vi "NI Camera Loop.vi"(6 "Used functions":bool=TRUE, 8 "error in":errorcluster, 9 "IBM OptoElectroMechanics Configuration":T1={"Parameter Analizer"={"Parameter Analyzer VISA Session"="COM1", "Sweeping Time Parameters"={"Integration Time"=0, "Short Integration Time (s)"=1.0, "Long Integration Time (s)"=0.0, "Wait Time Parameter"=1.0}, "Acquisition Mode"=enum."Sweeping Mode", "Status Polling Time (ms)"=0, "Comment"="Test VI", "SMU 1 - Sweeping"={"Start / Offset"=0.0, "Stop / Ratio"=1.0, "Step \n(linear only)"=0.01, "Compliance"=0.1, "Power \nCompliance"=0.0, "Mode"=0, "Function"=0, "Sweep Mode"=FALSE}, "SMU 2 - Sweeping"={"Start / Offset"=0.0, "Stop / Ratio"=1.0, "Step \n(linear only)"=0.01, "Compliance"=0.1, "Power \nCompliance"=0.0, "Mode"=0, "Function"=0, "Sweep Mode"=FALSE}, "SMU 3 - Sweeping"={"Start / Offset"=0.0, "Stop / Ratio"=1.0, "Step \n(linear only)"=0.01, "Compliance"=0.1, "Power \nCompliance"=0.0, "Mode"=0, "Function"=0, "Sweep Mode"=FALSE}, "SMU 4 - Sweeping"={"Start / Offset"=0.0, "Stop / Ratio"=1.0, "Step \n(linear only)"=0.01, "Compliance"=0.1, "Power \nCompliance"=0.0, "Mode"=0, "Function"=0, "Sweep Mode"=FALSE}, "Sweep Spacing"=0, "Range"=0, "SMU1 - Sampling"={"Source"=10.0, "Compliance"=1e-05, "Mode"=0, "Function"=FALSE}, "SMU2 - Sampling"={"Source"=1.0, "Compliance"=1.0, "Mode"=0, "Function"=FALSE}, "SMU3 - Sampling"={"Source"=10.0, "Compliance"=1e-05, "Mode"=0, "Function"=FALSE}, "SMU4 - Sampling"={"Source"=0.1, "Compliance"=60.0, "Mode"=10, "Function"=FALSE}, "Sampling Time Parameters"={"Initial Interval (s)"=0.1, "Number of Samples"=60, "Total Sampling Time (s)"=10.0, "Hold Time (s)"=0.0, "Sampling Mode"=0, "Sampling Time"=0}, "Stop Condition"={"Enable Delay (s)"=0.0, "Name"="", "Threshold"=0.0, "num. of events"=1, "Event"=0, "Stop Condition Enable"=FALSE}}, "Switching Matrix"={"Switching Matrix VISA Session"="GPIB0::18::INSTR", "Connections"=[{"Connections"=[FALSE, FALSE, FALSE, FALSE, FALSE, FALSE, FALSE, FALSE, FALSE, FALSE, FALSE, FALSE], "Connection Type"=enum."Disconnected"}, {"Connections"=[FALSE, FALSE, FALSE, FALSE, FALSE, FALSE, FALSE, FALSE, FALSE, FALSE, FALSE, FALSE], "Connection Type"=enum."Disconnected"}, {"Connections"=[FALSE, FALSE, FALSE, FALSE, FALSE, FALSE, FALSE, FALSE, FALSE, FALSE, FALSE, FALSE], "Connection Type"=enum."Disconnected"}, {"Connections"=[FALSE, FALSE, FALSE, FALSE, FALSE, FALSE, FALSE, FALSE, FALSE, FALSE, FALSE, FALSE], "Connection Type"=enum."Disconnected"}, {"Connections"=[FALSE, FALSE, FALSE, FALSE, FALSE, FALSE, FALSE, FALSE, FALSE, FALSE, FALSE, FALSE], "Connection Type"=enum."Disconnected"}, {"Connections"=[FALSE, FALSE, FALSE, FALSE, FALSE, FALSE, FALSE, FALSE, FALSE, FALSE, FALSE, FALSE], "Connection Type"=enum."Disconnected"}, {"Connections"=[FALSE, FALSE, FALSE, FALSE, FALSE, FALSE, FALSE, FALSE, FALSE, FALSE, FALSE, FALSE], "Connection Type"=enum."Disconnected"}, {"Connections"=[FALSE, FALSE, FALSE, FALSE, FALSE, FALSE, FALSE, FALSE, FALSE, FALSE, FALSE, FALSE], "Connection Type"=enum."Disconnected"}]}, "Stress Control"={"Stress Control VISA Session"="StrainMotor", "Axis"=0, "Motion"=0, "Destination (°)"=0.0, "Speed (°/s)"=4.0, "Position (°)"=25.0}, "Optical Spectrometer"={"Laser Settings"={"Laser Wavelength"=enum."365 nm", "Neutral Density Filter"=enum."100%"}, "Spectrometer Settings"={"Confocal Hole Size (µm)"=0.0, "Grating"=2, "Detector"=enum."InGaAs Array"}, "Acquisition Settings"={"Acquisition Mode"=enum."Multi-Window", "Spectal Position (nm)"=632.0, "From (nm)"=735.0, "To (nm)"=0.0, "Integration Time (s)"=0.0, "Number of Accumulations"=3, "AutoScanning"=FALSE, "Spike Removal"=FALSE}, "Path"=path "C:/07 - Prizes and Awards/Marie Curie Prize/Reply Editors Final NCOMMS(10).docx"}, "Switches & Mirrors"={"Relay VISA Session"="COM1", "Switches"={"Laser"=FALSE, "Video"=FALSE}, "Delays (ms)"={"Laser"=500, "Video"=1500}}, "Camera"={"Settings"={"Pixel clock"=20, "Frame rate"=30.0, "Exposure time"=33.21525, "Master Gain"=0, "Red Gain"=0, "Green Gain"=0, "Blue Gain"=0, "Auto Gain"=FALSE, "White-balance"=FALSE, "Color Correction"=FALSE}}, "XYZ Stage"={"Connection Settings"={"Tango VISA"="", "Baudrate"=57600, "Show Protocol?"=FALSE}, "Manual Control"={"North"=FALSE, "South"=FALSE, "West"=FALSE, "East"=FALSE, "Up"=FALSE, "Down"=FALSE, "Stop"=FALSE, "XY Step"=0.0, "Z step"=0.0}, "Coordinate Control"={"Motion Mode"=enum."Absolute", "Destination [mm]"=[]}}, "AutoFocus"={"Matching Criteria"={"Minimum Score"=700.0, "Color Score Weight"=700.0, "Minimum Contrast"=50, "Match Mode"=0, "Match Feature Mode"=0, "Subpixel Accuracy"=TRUE, "Color Sensitivity"=1, "Search Strategy"=1}, "Z Scan Parameters"={"Z Range"=1380.0, "Resolution"=5000.0, "Initial Direction"=enum."Up", "Focus Threshold"=0.1, "Ascent Constant"=0.1}, "Displacement"=0.0, "Transformation Matrix"=[]}, "Sava Data"={"Workspace Info"={"Device Name"="ProberHead_Tst_C29K3_7(2)", "Device Info"="ProberHead_Tst_C29", "Path"=path "C:/Users/gio/Desktop/ProbeHeadTest"}, "Instrument Configuration"={"Instrument"=enum."Unknown Instrument", "Configuration"="Test Configuration"}, "Stress Motor Position"=0.0, "Electrical Measurement"={"Sequence"=[], "V1"=[], "V2"=[], "V3"=[], "V4"=[], "I1"=[], "I2"=[], "I3"=[], "I4"=[]}, "Optical Spectrum"={"Intensity"=[], "Wavelength"=[], "Energy"=[], "Raman Shift"=[], "Detector Temperature"=0.0}}, "PlotData"={"Sliders"={"Strain Sequence"=0, "Instrument Sequence"=0}, "Measurement"={"Which Instrument?"=enum."No Plot", "Electrical Measurement"={"Sequence"=[], "V1"=[], "V2"=[], "V3"=[], "V4"=[], "I1"=[], "I2"=[], "I3"=[], "I4"=[]}, "Measurement Mode"=enum."Sweeping Mode", "Optical Spectrum"={"Intensity"=[], "Wavelength"=[], "Energy"=[], "Raman Shift"=[], "Detector Temperature"=0.0}}, "Instrument Steps"=[], "Strain Points"=[]}, "Instrument Sequence"={"Caller VI"=enum."User"}, "Strain Measurement"={"Stress Sequence "={"Max Motor Position"=1380.0, "# Intermediate Points"=5000, "Initial Direction"=enum."Tension"}, "Track?"=FALSE}} {"AutoFocus"."Displacement" scale=1.0..1000.0; "AutoFocus"."Z Scan Parameters"."Focus Threshold" min=0.0 max=1000.0 step=1.0 format="%#_2f"; "AutoFocus"."Z Scan Parameters"."Ascent Constant" min=0.0 max=1000.0 step=1.0 format="%#_2f"; "AutoFocus"."Z Scan Parameters"."Resolution" min=0.0 max=1.0 step=0.01 format="%_2g"; "AutoFocus"."Z Scan Parameters"."Z Range" format="%_3g"; "AutoFocus"."Matching Criteria"."Match Mode" items=["Shift Invariant", "Rotation Invariant"]; "AutoFocus"."Matching Criteria"."Match Feature Mode" items=["Color and Shape", "Color", "Shape"]; "AutoFocus"."Matching Criteria"."Color Sensitivity" items=["Low Sensitivity", "Medium Sensitivity", "High Sensitivity"]; "AutoFocus"."Matching Criteria"."Search Strategy" items=["Conservative", "Balance", "Aggressive", "Very Aggressive"]; "XYZ Stage"."Manual Control"."Z step" scale=0.1..10.0; "XYZ Stage"."Manual Control"."XY Step" scale=0.1..1000.0; "Camera"."Settings"."Blue Gain" min=0 max=100 scale=0.0..100.0; "Camera"."Settings"."Green Gain" min=0 max=100 scale=0.0..100.0; "Camera"."Settings"."Red Gain" min=0 max=100 scale=0.0..100.0; "Camera"."Settings"."Master Gain" min=0 max=100 scale=0.0..100.0; "Camera"."Settings"."Exposure time" min=0.101625 max=159.246375 step=0.101625 scale=0.101625..159.246375 scale format="%#.3g"; "Camera"."Settings"."Frame rate" min=2.7455631699174137 max=6.2675785993528725 step=0.000101625 scale=2.7455631699174137..6.2675785993528725 scale format="%^#_3g"; "Camera"."Settings"."Pixel clock" min=5 max=43 scale=5.0..43.0; "PlotData"."Sliders"."Instrument Sequence" scale=0.0..10.0; "PlotData"."Sliders"."Strain Sequence" scale=0.0..10.0; "Strain Measurement"."Stress Sequence"."# Intermediate Points" max=1390; "Parameter Analizer"."Stop Condition"."Event" items=["Value > Threshold", "Value < Threshold", "| Value | > | Threshold |", "| Value | < | Threshold |"]; "Parameter Analizer"."Stop Condition"."Threshold" format="%^.2e"; "Parameter Analizer"."Stop Condition"."Enable Delay (s)" format="%.1f"; "Parameter Analizer"."Sampling Time Parameters"."Sampling Time" items=["Auto (linear only)", "No Limit", "Set Limit"]; "Parameter Analizer"."Sampling Time Parameters"."Sampling Mode" items=["Linear", "Log10", "Log25", "Log50", "Thinned Out"]; "Parameter Analizer"."Sampling Time Parameters"."Hold Time (s)" format="%.4f"; "Parameter Analizer"."Sampling Time Parameters"."Total Sampling Time (s)" format="%.1f"; "Parameter Analizer"."Sampling Time Parameters"."Initial Interval (s)" format="%^.3e"; "Parameter Analizer"."SMU 4 - Sweeping"."Function" items=["Disabled", "Var 1", "Var 2", "Var 1'", "Constant"]; "Parameter Analizer"."SMU 4 - Sweeping"."Mode" items=["V", "I", "V pulse", "I  pulse", "Common"]; "Parameter Analizer"."SMU 4 - Sweeping"."Power \nCompliance" format="%^.2e"; "Parameter Analizer"."SMU 4 - Sweeping"."Compliance" format="%^.2e"; "Parameter Analizer"."SMU 4 - Sweeping"."Step \n(linear only)" format="%^.4e"; "Parameter Analizer"."SMU 4 - Sweeping"."Stop / Ratio" format="%^.4e"; "Parameter Analizer"."SMU 4 - Sweeping"."Start / Offset" format="%^.4e"; "Parameter Analizer"."SMU 3 - Sweeping"."Function" items=["Disabled", "Var 1", "Var 2", "Var 1'", "Constant"]; "Parameter Analizer"."SMU 3 - Sweeping"."Mode" items=["V", "I", "V pulse", "I  pulse", "Common"]; "Parameter Analizer"."SMU 3 - Sweeping"."Power \nCompliance" format="%^.2e"; "Parameter Analizer"."SMU 3 - Sweeping"."Compliance" format="%^.2e"; "Parameter Analizer"."SMU 3 - Sweeping"."Step \n(linear only)" format="%^.4e"; "Parameter Analizer"."SMU 3 - Sweeping"."Stop / Ratio" format="%^.4e"; "Parameter Analizer"."SMU 3 - Sweeping"."Start / Offset" format="%^.4e"; "Parameter Analizer"."SMU 2 - Sweeping"."Function" items=["Disabled", "Var 1", "Var 2", "Var 1'", "Constant"]; "Parameter Analizer"."SMU 2 - Sweeping"."Mode" items=["V", "I", "V pulse", "I  pulse", "Common"]; "Parameter Analizer"."SMU 2 - Sweeping"."Power \nCompliance" format="%^.2e"; "Parameter Analizer"."SMU 2 - Sweeping"."Compliance" format="%^.2e"; "Parameter Analizer"."SMU 2 - Sweeping"."Step \n(linear only)" format="%^.4e"; "Parameter Analizer"."SMU 2 - Sweeping"."Stop / Ratio" format="%^.4e"; "Parameter Analizer"."SMU 2 - Sweeping"."Start / Offset" format="%^.4e"; "Parameter Analizer"."SMU 1 - Sweeping"."Function" items=["Disabled", "Var 1", "Var 2", "Var 1'", "Constant"]; "Parameter Analizer"."SMU 1 - Sweeping"."Mode" items=["V", "I", "V pulse", "I  pulse", "Common"]; "Parameter Analizer"."SMU 1 - Sweeping"."Power \nCompliance" format="%^.2e"; "Parameter Analizer"."SMU 1 - Sweeping"."Compliance" format="%^.2e"; "Parameter Analizer"."SMU 1 - Sweeping"."Step \n(linear only)" format="%^.4e"; "Parameter Analizer"."SMU 1 - Sweeping"."Stop / Ratio" format="%^.4e"; "Parameter Analizer"."SMU 1 - Sweeping"."Start / Offset" format="%^.4e"; "Parameter Analizer"."Sweeping Time Parameters"."Long Integration Time (s)" scale=0.02..2.0; "Parameter Analizer"."Sweeping Time Parameters"."Short Integration Time (s)" scale=8e-05..0.00192; "Parameter Analizer"."Sweeping Time Parameters"."Integration Time" items=["Short", "Long"]; "Parameter Analizer"."Sweeping Time Parameters"."Wait Time Parameter" format="%.1f"; "Parameter Analizer"."SMU4 - Sampling"."Mode" items=["V", "I", "Common"]; "Parameter Analizer"."SMU4 - Sampling"."Compliance" format="%^.2e"; "Parameter Analizer"."SMU4 - Sampling"."Source" format="%^.3e"; "Parameter Analizer"."SMU3 - Sampling"."Mode" items=["V", "I", "Common"]; "Parameter Analizer"."SMU3 - Sampling"."Compliance" format="%^.2e"; "Parameter Analizer"."SMU3 - Sampling"."Source" format="%^.3e"; "Parameter Analizer"."SMU2 - Sampling"."Mode" items=["V", "I", "Common"]; "Parameter Analizer"."SMU2 - Sampling"."Compliance" format="%^.2e"; "Parameter Analizer"."SMU2 - Sampling"."Source" format="%^.3e"; "Parameter Analizer"."SMU1 - Sampling"."Mode" items=["V", "I", "Common"]; "Parameter Analizer"."SMU1 - Sampling"."Compliance" format="%^.2e"; "Parameter Analizer"."SMU1 - Sampling"."Source" format="%^.3e"; "Parameter Analizer"."Range" items=["auto", "fixed", "limited"]; "Parameter Analizer"."Sweep Spacing" items=["linear", "log 10", "log 25", "log 50"]; "Stress Control"."Axis" min=1 max=3; "Stress Control"."Position (°)" format="%.6g"; "Stress Control"."Speed (°/s)" min=0.0 max=4.0 format="%.6f"; "Stress Control"."Destination (°)" min=-2000000000.0 max=2000000000.0 format="%.6f"; "Stress Control"."Motion" items=["Absolute", "Relative"]; "Optical Spectrometer"."Spectrometer Settings"."Grating" items=["1800 l/mm", "150 l/mm"]}, 10 "Message Queues out":T57, 11 "Notifiers":T44) -> (0 "error out":errorcluster)   [LabVIEW 2014]
uses:
  support/Message Queue/All Message Queues.ctl
  support/Message Queue/Message Cluster.ctl
  support/Notifiers/Notifiers.ctl
  support/Message Handler Loop Notifiers.ctl
  Hardware Control/Parameter Analyzer/Parameter Analyzer Notifiers.ctl
  Hardware Control/Switching Matrix/Switching Matrix Notifiers.ctl
  Hardware Control/Stress Control/StressControl Notifiers.ctl
  Hardware Control/Spectrometer/Spectrometer Notifiers.ctl
  Hardware Control/Switches and Mirrors/SwitchesMirrors Notifiers.ctl
  Hardware Control/Camera/Camera Notifiers.ctl
  Hardware Control/XYZ Stage/XYZ Notifications.ctl
  Hardware Control/Autofocus/Autofocus Notifiers.ctl
  Measurements/Optoelectronic Measurement/Optoelectronic Notifiers.ctl
  Measurements/Save Data/SaveData Notifiers.ctl
  Measurements/Instrument Sequence/Instrument Sequence Notifiers.ctl
  support/Configuration/Configuration.ctl
  Hardware Control/Parameter Analyzer/Parameter Analyzer Config.ctl
  Hardware Control/Parameter Analyzer/Parameter Analyzer Integration Parameters.ctl
  Hardware Control/Parameter Analyzer/Parameter Analyzer SMU Sweeping.ctl
  Hardware Control/Parameter Analyzer/Parameter Analyzer Sweep Spacing.ctl
  Hardware Control/Parameter Analyzer/Parameter Analyzer SMU Range.ctl
  Hardware Control/Parameter Analyzer/Parameter Analyzer SMU Sampling.ctl
  Hardware Control/Parameter Analyzer/Parameter Analyzer Sampling Parameters.ctl
  Hardware Control/Parameter Analyzer/Parameter Analyzer Stop Sampling Conditions.ctl
  Hardware Control/Switching Matrix/Switching Matrix Config.ctl
  Hardware Control/Stress Control/StressControl Config.ctl
  Hardware Control/Spectrometer/Spectrometer Config.ctl
  Hardware Control/Spectrometer/Laser Settings.ctl
  Hardware Control/Spectrometer/Laser.ctl
  Hardware Control/Spectrometer/Filter.ctl
  Hardware Control/Spectrometer/Grating Detector Settings.ctl
  Hardware Control/Spectrometer/Grating.ctl
  Hardware Control/Spectrometer/Detector.ctl
  Hardware Control/Spectrometer/Acquisition Settings.ctl
  Hardware Control/Switches and Mirrors/SwitchesMirrors Config.ctl
  Hardware Control/Switches and Mirrors/SwitchesMirrors Status.ctl
  Hardware Control/Camera/Camera Config.ctl
  Hardware Control/Camera/Camera Settings.ctl
  Hardware Control/XYZ Stage/XYZ Config.ctl
  Hardware Control/XYZ Stage/XYZ Connection Settings.ctl
  Hardware Control/XYZ Stage/XYZ Stage Control.ctl
  Hardware Control/XYZ Stage/XYZ Coordinate Control.ctl
  Hardware Control/Autofocus/AutoFocus Config.ctl
  Hardware Control/Autofocus/ZScan.ctl
  <vilib>/Analysis/Matrix/Datatypes/RealMatrix.ctl
  Measurements/Save Data/SaveData Config.ctl
  Measurements/Save Data/SaveData Workspace Info.ctl
  Measurements/Save Data/SaveData Instrument Configuration.ctl
  Measurements/Instrument Sequence/Instrument List.ctl
  Hardware Control/Spectrometer/Spectral Data.ctl
  Measurements/Plot Data/PlotData Config.ctl
  Measurements/Plot Data/Measurement.ctl
  Measurements/Plot Data/WhichInstrument.ctl
  Hardware Control/Parameter Analyzer/Electrical Data.ctl
  Measurements/Instrument Sequence/Instrument Steps.ctl
  Measurements/Instrument Sequence/Action.ctl
  Measurements/Instrument Sequence/Instrument Sequence Config.ctl
  Measurements/Strain Measurement/Strain Measurement Config.ctl
  Hardware Control/Camera/NI Camera Functions.ctl
  support/Message Queue/Message Queue.lvlib
  <vilib>/Analysis/Matrix/NI_Matrix.lvlib
panel:
  # "LICENSED MATERIALS – PROPERTY OF IBM\nCopyright IBM Corp. 2016,\nALL RIGHTS RESERVED"
  # "XY"
  # "Z"
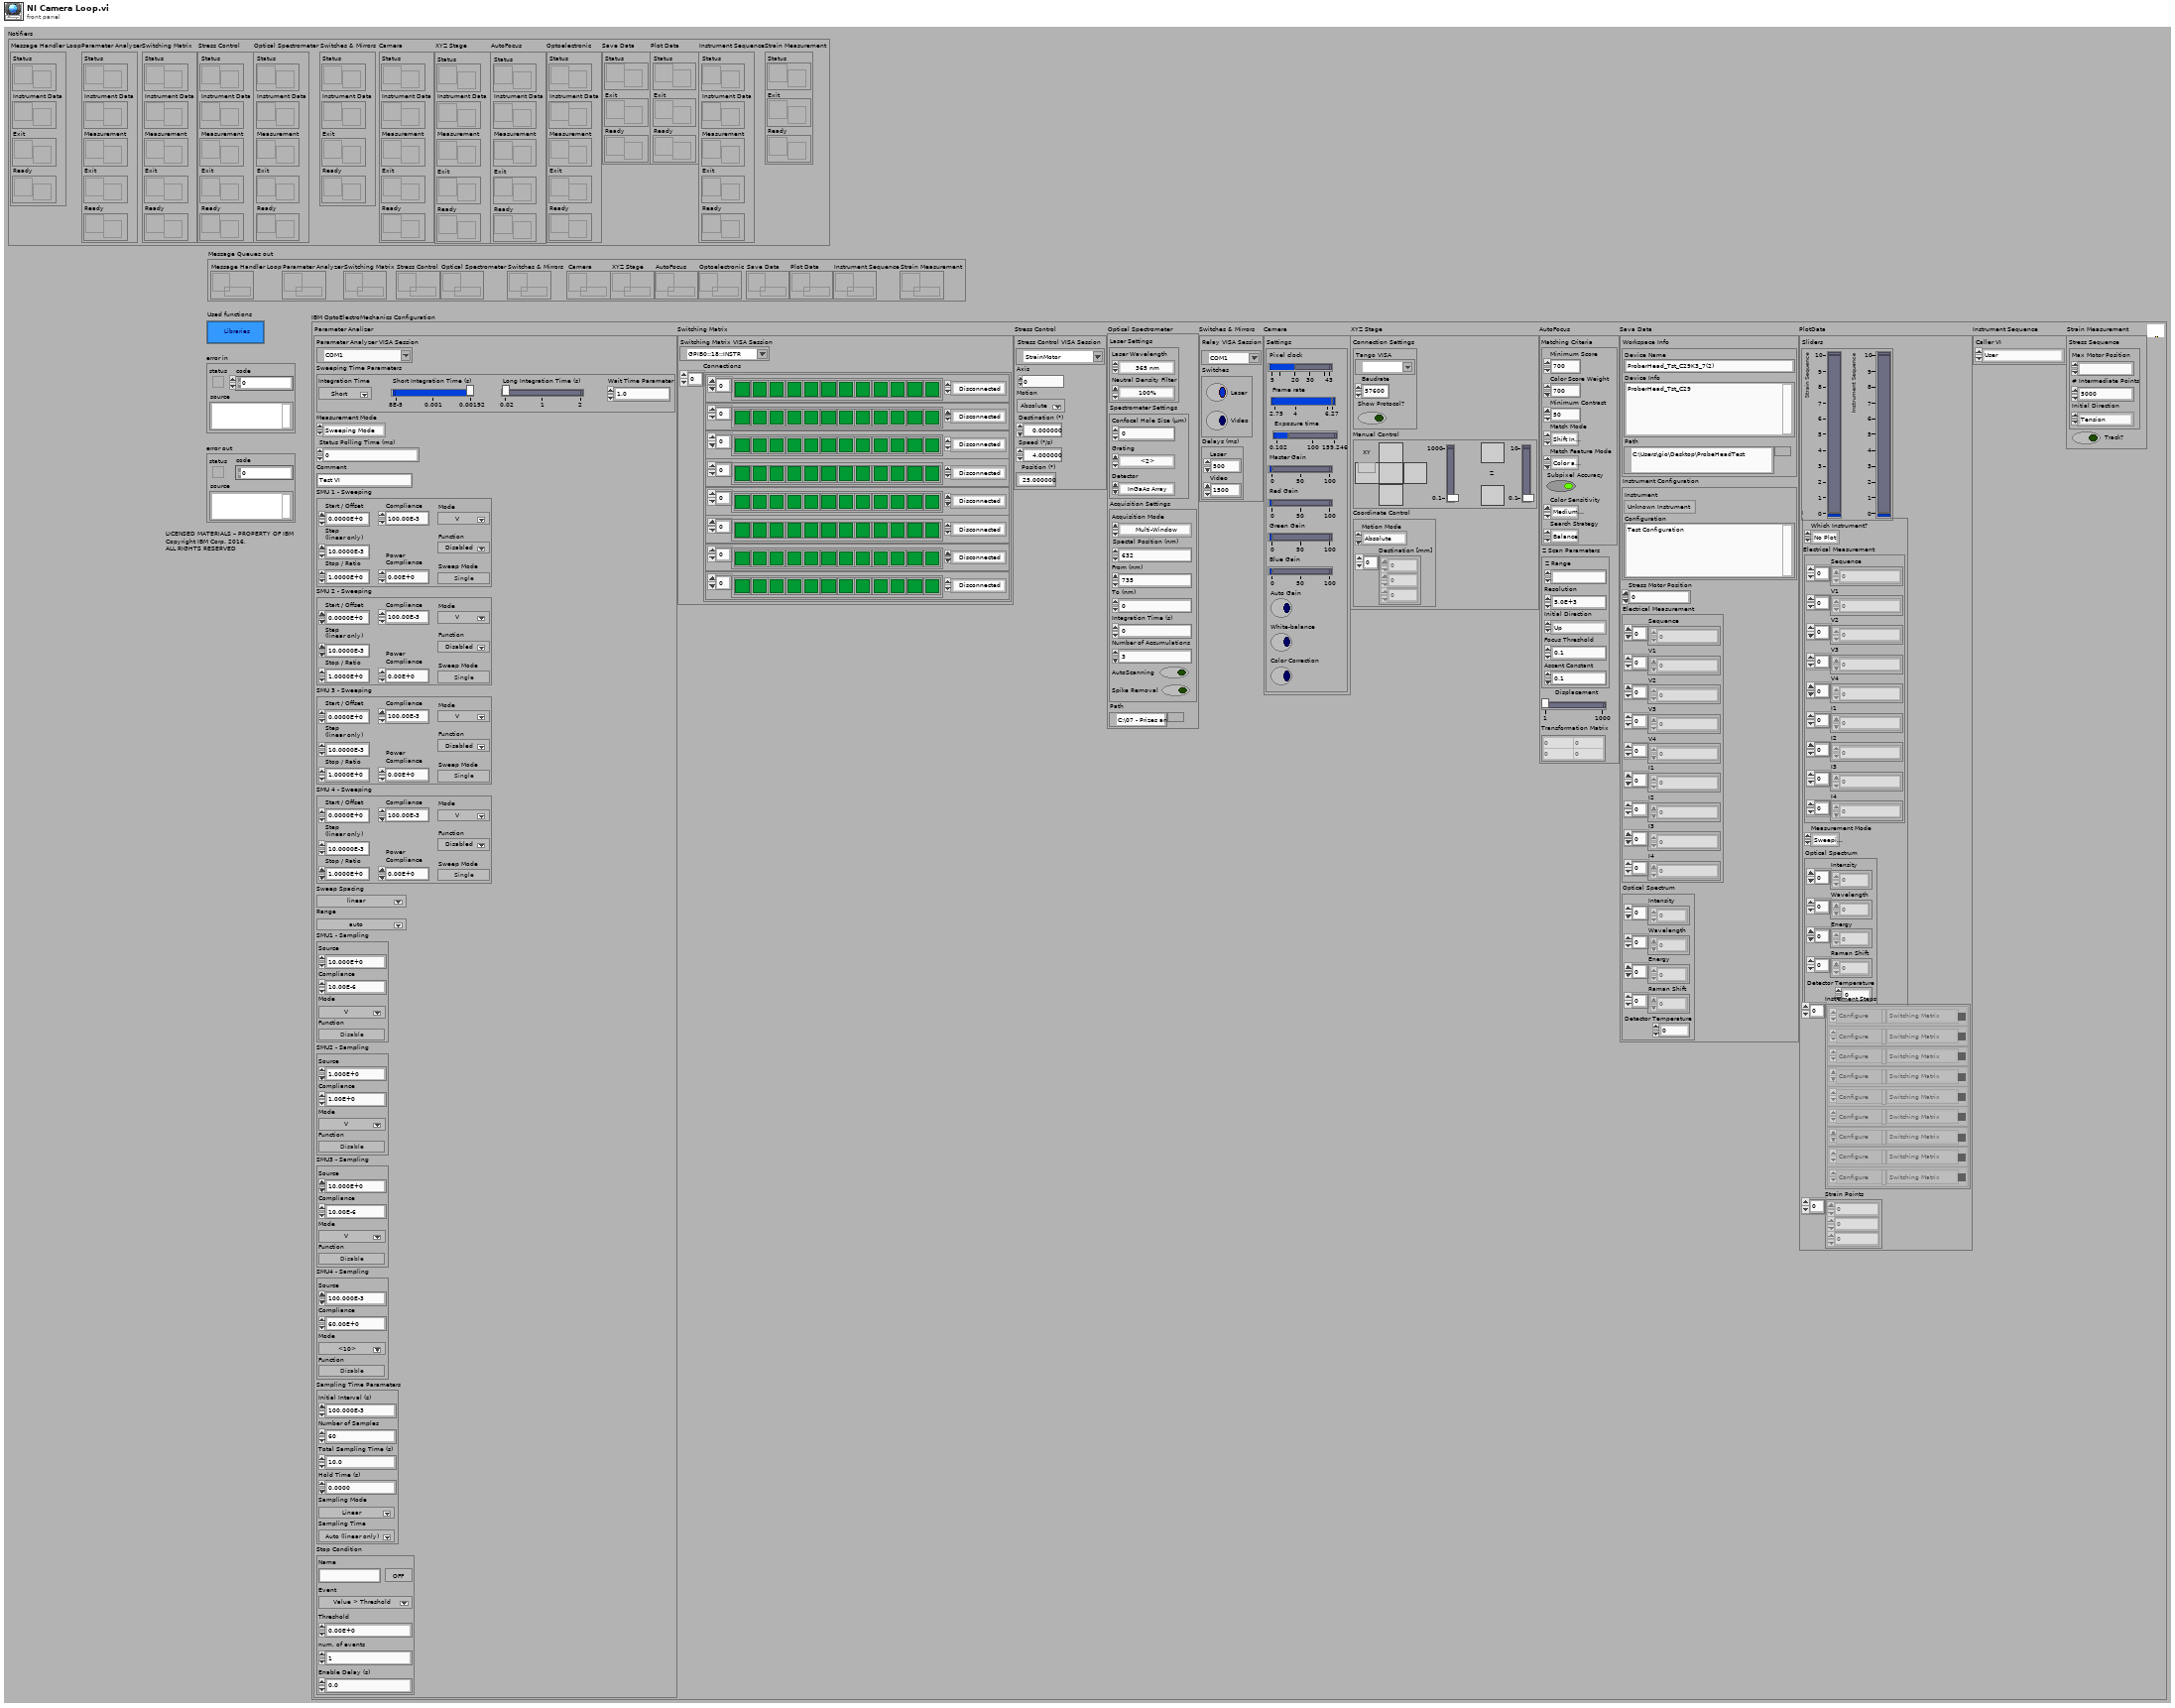
[diagram p1: front panel]
types:
  T1 = typedef "Configuration.ctl" = cluster{"Parameter Analizer":T2, "Switching Matrix":T10, "Stress Control":T11, "Optical Spectrometer":T12, "Switches & Mirrors":T20, "Camera":T22, "XYZ Stage":T24, "AutoFocus":T28, "Sava Data":T31, "PlotData":T36, "Instrument Sequence":T42, "Strain Measurement":T43}
  T2 = typedef "Parameter Analyzer Config.ctl" = cluster{"Parameter Analyzer VISA Session":refnum<visa-resource-name>, "Sweeping Time Parameters":T3, "Acquisition Mode":enum32{"Sweeping Mode", "Sampling Mode"}, "Status Polling Time (ms)":u32, "Comment":string, "SMU 1 - Sweeping":T4, "SMU 2 - Sweeping":T4, "SMU 3 - Sweeping":T4, "SMU 4 - Sweeping":T4, "Sweep Spacing":T5, "Range":T6, "SMU1 - Sampling":T7, "SMU2 - Sampling":T7, "SMU3 - Sampling":T7, "SMU4 - Sampling":T7, "Sampling Time Parameters":T8, "Stop Condition":T9}
  T3 = typedef "Parameter Analyzer Integration Parameters.ctl" = cluster{"Integration Time":u32, "Short Integration Time (s)":dbl, "Long Integration Time (s)":dbl, "Wait Time Parameter":dbl}
  T4 = typedef "Parameter Analyzer SMU Sweeping.ctl" = cluster{"Start / Offset":dbl, "Stop / Ratio":dbl, "Step \n(linear only)":dbl, "Compliance":dbl, "Power \nCompliance":dbl, "Mode":u32, "Function":i32, "Sweep Mode":bool}
  T5 = typedef "Parameter Analyzer Sweep Spacing.ctl" = u16
  T6 = typedef "Parameter Analyzer SMU Range.ctl" = u16
  T7 = typedef "Parameter Analyzer SMU Sampling.ctl" = cluster{"Source":dbl, "Compliance":dbl, "Mode":u32, "Function":bool}
  T8 = typedef "Parameter Analyzer Sampling Parameters.ctl" = cluster{"Initial Interval (s)":dbl, "Number of Samples":i32, "Total Sampling Time (s)":dbl, "Hold Time (s)":dbl, "Sampling Mode":i32, "Sampling Time":i32}
  T9 = typedef "Parameter Analyzer Stop Sampling Conditions.ctl" = cluster{"Enable Delay (s)":dbl, "Name":string, "Threshold":dbl, "num. of events":i32, "Event":i32, "Stop Condition Enable":bool}
  T10 = typedef "Switching Matrix Config.ctl" = cluster{"Switching Matrix VISA Session":refnum<visa-resource-name>, "Connections":cluster{"Connections":bool[], "Connection Type":enum16{"Disconnected", "Make - Break", "Break - Make"}}[]}
  T11 = typedef "StressControl Config.ctl" = cluster{"Stress Control VISA Session":refnum<visa-resource-name>, "Axis":i32, "Motion":u16, "Destination (°)":dbl, "Speed (°/s)":dbl, "Position (°)":dbl}
  T12 = typedef "Spectrometer Config.ctl" = cluster{"Laser Settings":T13, "Spectrometer Settings":T16, "Acquisition Settings":T19, "Path":path}
  T13 = typedef "Laser Settings.ctl" = cluster{"Laser Wavelength":T14, "Neutral Density Filter":T15}
  T14 = typedef "Laser.ctl" = enum16{"633 nm", "784 nm", "532 nm", "365 nm"}
  T15 = typedef "Filter.ctl" = enum16{"100%", "50%", "25%", "10%", "1%", "0.1%", "0.01%"}
  T16 = typedef "Grating Detector Settings.ctl" = cluster{"Confocal Hole Size (µm)":dbl, "Grating":T17, "Detector":T18}
  T17 = typedef "Grating.ctl" = u16
  T18 = typedef "Detector.ctl" = enum16{"InGaAs Array", "Silicon CCD"}
  T19 = typedef "Acquisition Settings.ctl" = cluster{"Acquisition Mode":enum16{"Single Window", "Multi-Window"}, "Spectal Position (nm)":dbl, "From (nm)":dbl, "To (nm)":dbl, "Integration Time (s)":dbl, "Number of Accumulations":i32, "AutoScanning":bool, "Spike Removal":bool}
  T20 = typedef "SwitchesMirrors Config.ctl" = cluster{"Relay VISA Session":refnum<visa-resource-name>, "Switches":T21, "Delays (ms)":cluster{"Laser":u32, "Video":u32}}
  T21 = typedef "SwitchesMirrors Status.ctl" = cluster{"Laser":bool, "Video":bool}
  T22 = typedef "Camera Config.ctl" = cluster{"Settings":T23}
  T23 = typedef "Camera Settings.ctl" = cluster{"Pixel clock":i32, "Frame rate":dbl, "Exposure time":dbl, "Master Gain":i32, "Red Gain":i32, "Green Gain":i32, "Blue Gain":i32, "Auto Gain":bool, "White-balance":bool, "Color Correction":bool}
  T24 = typedef "XYZ Config.ctl" = cluster{"Connection Settings":T25, "Manual Control":T26, "Coordinate Control":T27}
  T25 = typedef "XYZ Connection Settings.ctl" = cluster{"Tango VISA":refnum<visa-resource-name>, "Baudrate":i32, "Show Protocol?":bool}
  T26 = typedef "XYZ Stage Control.ctl" = cluster{"North":bool, "South":bool, "West":bool, "East":bool, "Up":bool, "Down":bool, "Stop":bool, "XY Step":dbl, "Z step":dbl}
  T27 = typedef "XYZ Coordinate Control.ctl" = cluster{"Motion Mode":enum16{"Absolute", "Relative"}, "Destination [mm]":dbl[]}
  T28 = typedef "AutoFocus Config.ctl" = cluster{"Matching Criteria":cluster{"Minimum Score":sgl, "Color Score Weight":sgl, "Minimum Contrast":i32, "Match Mode":u32, "Match Feature Mode":u32, "Subpixel Accuracy":bool, "Color Sensitivity":u32, "Search Strategy":u32}, "Z Scan Parameters":T29, "Displacement":dbl, "Transformation Matrix":T30}
  T29 = typedef "ZScan.ctl" = cluster{"Z Range":ext, "Resolution":dbl, "Initial Direction":enum16{"Up", "Down"}, "Focus Threshold":dbl, "Ascent Constant":dbl}
  T30 = typedef "NI_Matrix.lvlib/RealMatrix.ctl" = dbl[][]
  T31 = typedef "SaveData Config.ctl" = cluster{"Workspace Info":T32, "Instrument Configuration":T33, "Stress Motor Position":dbl, "Electrical Measurement":cluster{"Sequence":dbl[], "V1":dbl[], "V2":dbl[], "V3":dbl[], "V4":dbl[], "I1":dbl[], "I2":dbl[], "I3":dbl[], "I4":dbl[]}, "Optical Spectrum":T35}
  T32 = typedef "SaveData Workspace Info.ctl" = cluster{"Device Name":string, "Device Info":string, "Path":path}
  T33 = typedef "SaveData Instrument Configuration.ctl" = cluster{"Instrument":T34, "Configuration":string}
  T34 = typedef "Instrument List.ctl" = enum32{"Unknown Instrument", "Switching Matrix", "Parameter Analyzer", "Optical Spectrometer", "Optoelectronic", "Autofocus"}
  T35 = typedef "Spectral Data.ctl" = cluster{"Intensity":dbl[], "Wavelength":dbl[], "Energy":dbl[], "Raman Shift":dbl[], "Detector Temperature":dbl}
  T36 = typedef "PlotData Config.ctl" = cluster{"Sliders":cluster{"Strain Sequence":i32, "Instrument Sequence":i32}, "Measurement":T37, "Instrument Steps":T40, "Strain Points":dbl[]}
  T37 = typedef "Measurement.ctl" = cluster{"Which Instrument?":T38, "Electrical Measurement":T39, "Measurement Mode":enum16{"Sweeping Mode", "Sampling Mode"}, "Optical Spectrum":T35}
  T38 = typedef "WhichInstrument.ctl" = enum16{"No Plot", "Spectrometer", "Parameter Analyzer", "Optoelectronic"}
  T39 = typedef "Electrical Data.ctl" = cluster{"Sequence":dbl[], "V1":dbl[], "V2":dbl[], "V3":dbl[], "V4":dbl[], "I1":dbl[], "I2":dbl[], "I3":dbl[], "I4":dbl[]}
  T40 = typedef "Instrument Steps.ctl" = cluster{"Action":T41, "Configuration":variant, "Instrument":T34, "Status":enum8{"False", "True", "Mixed"}}[]
  T41 = typedef "Action.ctl" = enum32{"Configure", "Measure"}
  T42 = typedef "Instrument Sequence Config.ctl" = cluster{"Caller VI":enum16{"User", "Stress Measurement VI"}}
  T43 = typedef "Strain Measurement Config.ctl" = cluster{"Stress Sequence ":cluster{"Max Motor Position":ext, "# Intermediate Points":u32, "Initial Direction":enum16{"Tension", "Compression"}}, "Track?":bool}
  T44 = typedef "Notifiers.ctl" = cluster{"Message Handler Loop":T45, "Parameter Analyzer":T46, "Switching Matrix":T47, "Stress Control":T48, "Optical Spectrometer":T49, "Switches & Mirrors":T50, "Camera":T51, "XYZ Stage":T52, "AutoFocus":T53, "Optoelectronic":T54, "Save Data":T55, "Plot Data":T55, "Instrument Sequence":T56, "Strain Measurement":cluster{"Status":refnum<notifier>, "Exit":refnum<notifier>, "Ready":refnum<notifier>}}
  T45 = typedef "Message Handler Loop Notifiers.ctl" = cluster{"Status":refnum<notifier>, "Instrument Data":refnum<notifier>, "Exit":refnum<notifier>, "Ready":refnum<notifier>}
  T46 = typedef "Parameter Analyzer Notifiers.ctl" = cluster{"Status":refnum<notifier>, "Instrument Data":refnum<notifier>, "Measurement":refnum<notifier>, "Exit":refnum<notifier>, "Ready":refnum<notifier>}
  T47 = typedef "Switching Matrix Notifiers.ctl" = cluster{"Status":refnum<notifier>, "Instrument Data":refnum<notifier>, "Measurement":refnum<notifier>, "Exit":refnum<notifier>, "Ready":refnum<notifier>}
  T48 = typedef "StressControl Notifiers.ctl" = cluster{"Status":refnum<notifier>, "Instrument Data":refnum<notifier>, "Measurement":refnum<notifier>, "Exit":refnum<notifier>, "Ready":refnum<notifier>}
  T49 = typedef "Spectrometer Notifiers.ctl" = cluster{"Status":refnum<notifier>, "Instrument Data":refnum<notifier>, "Measurement":refnum<notifier>, "Exit":refnum<notifier>, "Ready":refnum<notifier>}
  T50 = typedef "SwitchesMirrors Notifiers.ctl" = cluster{"Status":refnum<notifier>, "Instrument Data":refnum<notifier>, "Exit":refnum<notifier>, "Ready":refnum<notifier>}
  T51 = typedef "Camera Notifiers.ctl" = cluster{"Status":refnum<notifier>, "Instrument Data":refnum<notifier>, "Measurement":refnum<notifier>, "Exit":refnum<notifier>, "Ready":refnum<notifier>}
  T52 = typedef "XYZ Notifications.ctl" = cluster{"Status":refnum<notifier>, "Instrument Data":refnum<notifier>, "Measurement":refnum<notifier>, "Exit":refnum<notifier>, "Ready":refnum<notifier>}
  T53 = typedef "Autofocus Notifiers.ctl" = cluster{"Status":refnum<notifier>, "Instrument Data":refnum<notifier>, "Measurement":refnum<notifier>, "Exit":refnum<notifier>, "Ready":refnum<notifier>}
  T54 = typedef "Optoelectronic Notifiers.ctl" = cluster{"Status":refnum<notifier>, "Instrument Data":refnum<notifier>, "Measurement":refnum<notifier>, "Exit":refnum<notifier>, "Ready":refnum<notifier>}
  T55 = typedef "SaveData Notifiers.ctl" = cluster{"Status":refnum<notifier>, "Exit":refnum<notifier>, "Ready":refnum<notifier>}
  T56 = typedef "Instrument Sequence Notifiers.ctl" = cluster{"Status":refnum<notifier>, "Instrument Data":refnum<notifier>, "Measurement":refnum<notifier>, "Exit":refnum<notifier>, "Ready":refnum<notifier>}
  T57 = typedef "Message Queue.lvlib/All Message Queues.ctl" = cluster{"Message Handler Loop":refnum<queue>, "Parameter Analyzer":refnum<queue>, "Switching Matrix":refnum<queue>, "Stress Control":refnum<queue>, "Optical Spectrometer":refnum<queue>, "Switches & Mirrors":refnum<queue>, "Camera":refnum<queue>, "XYZ Stage":refnum<queue>, "AutoFocus":refnum<queue>, "Optoelectronic":refnum<queue>, "Save Data":refnum<queue>, "Plot Data":refnum<queue>, "Instrument Sequence":refnum<queue>, "Strain Measurement":refnum<queue>}
  T58 = typedef "Camera Data.ctl" = cluster{"Configuration":T22, "Refnums":T59, "Initialization":T60}
  T59 = typedef "Camera Refnums.ctl" = cluster{"Pixel Clock":refnum<vi>, "Frame Rate":refnum<vi>, "Exposure Time":refnum<vi>, "Master Gain":refnum<vi>, "Red Gain":refnum<vi>, "Green Gain":refnum<vi>, "Blue Gain":refnum<vi>, "Auto Gain":refnum<vi>, "Auto White-balance":refnum<vi>, "Color Correction":refnum<vi>, "Image":refnum<vi>, "Video Button":refnum<vi>, "Instrument Status":refnum<vi>}
  T60 = typedef "Camera Initialization.ctl" = cluster{"Connect":bool, "Update Refnums":bool, "Acquiring?":bool}
  T61 = typedef "NI Camera Functions.ctl" = enum16{"Connect", "Disconnect", "Start Live", "Stop Live", "Acquire", "Update Refnums"}
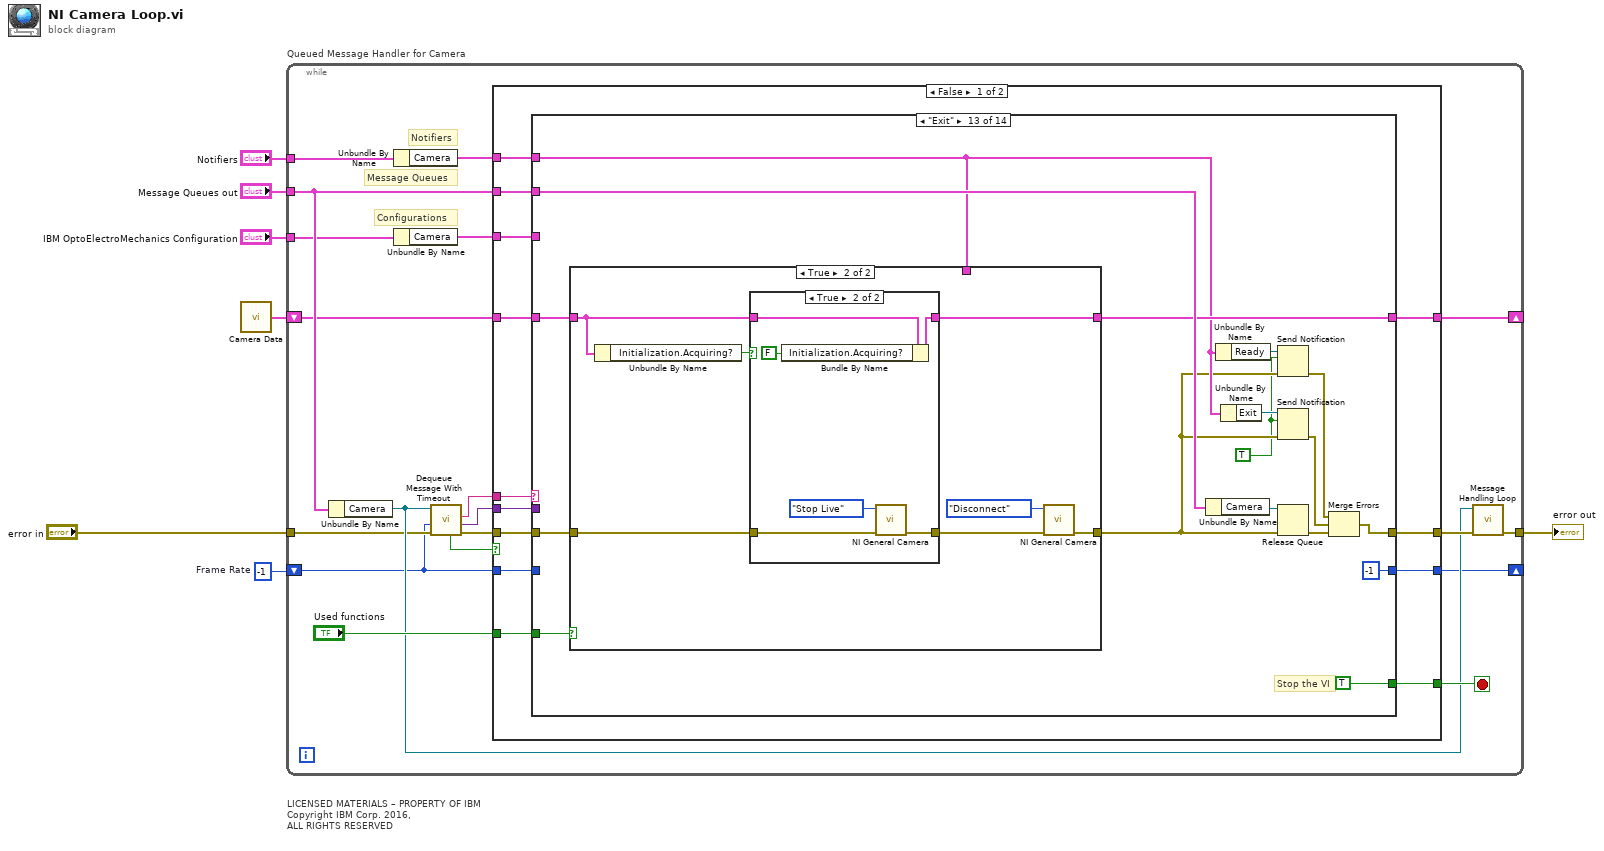
[diagram p0: block diagram]
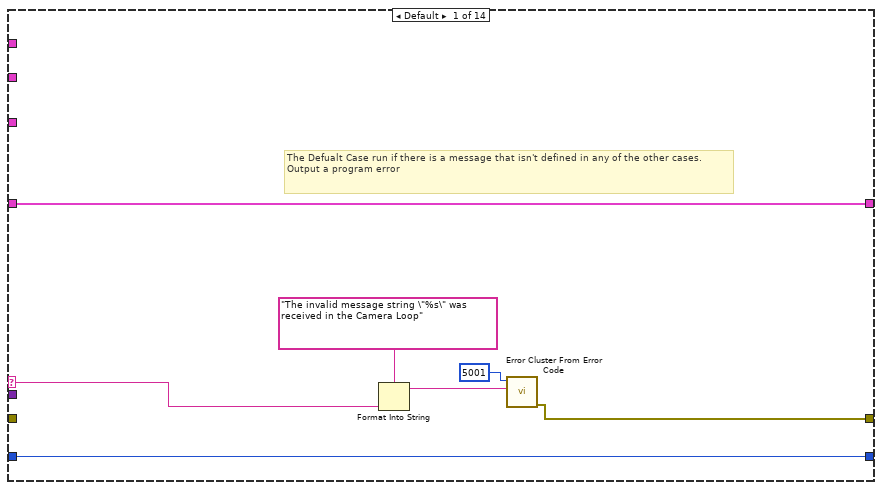
[diagram p2: hidden frame]
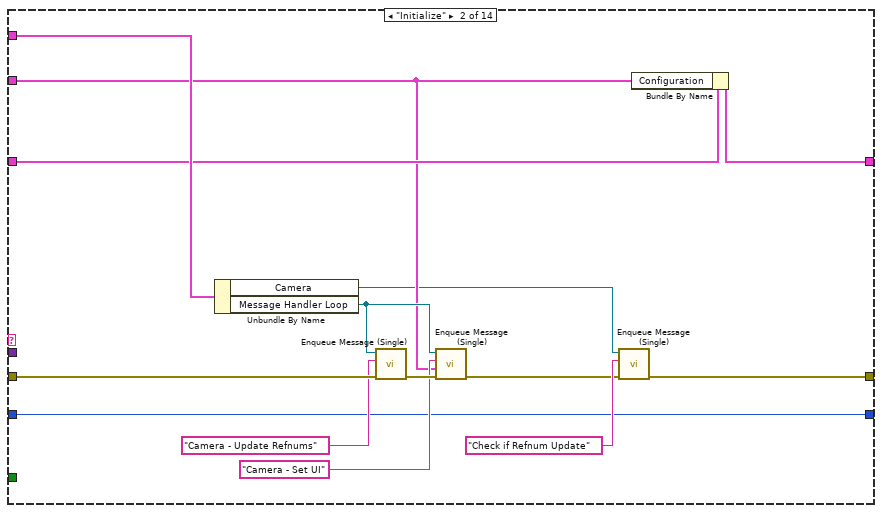
[diagram p3: hidden frame]
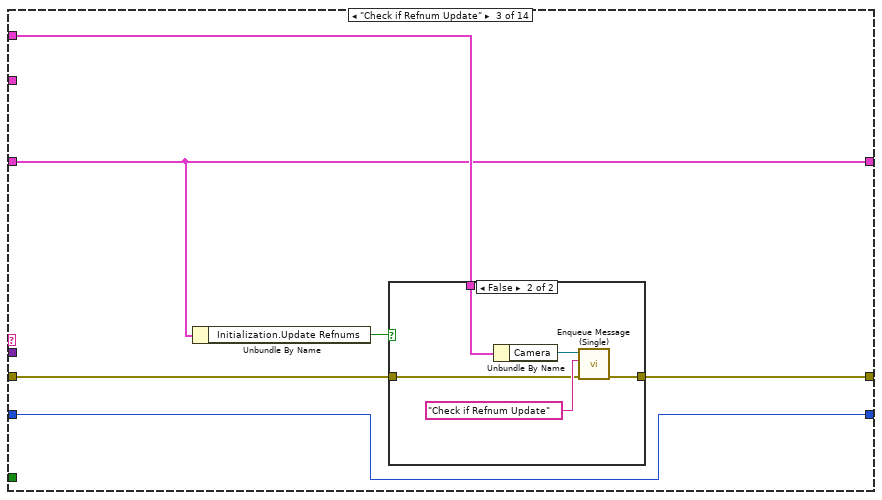
[diagram p4: hidden frame]
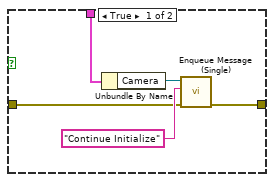
[diagram p5: hidden frame]
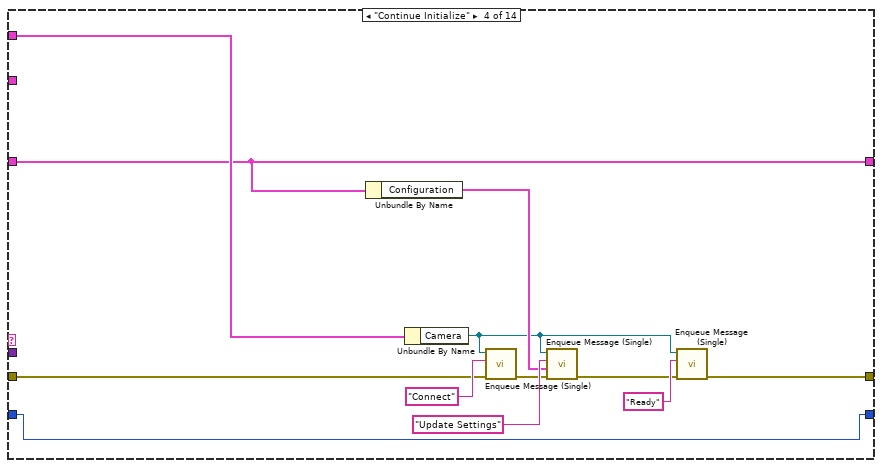
[diagram p6: hidden frame]
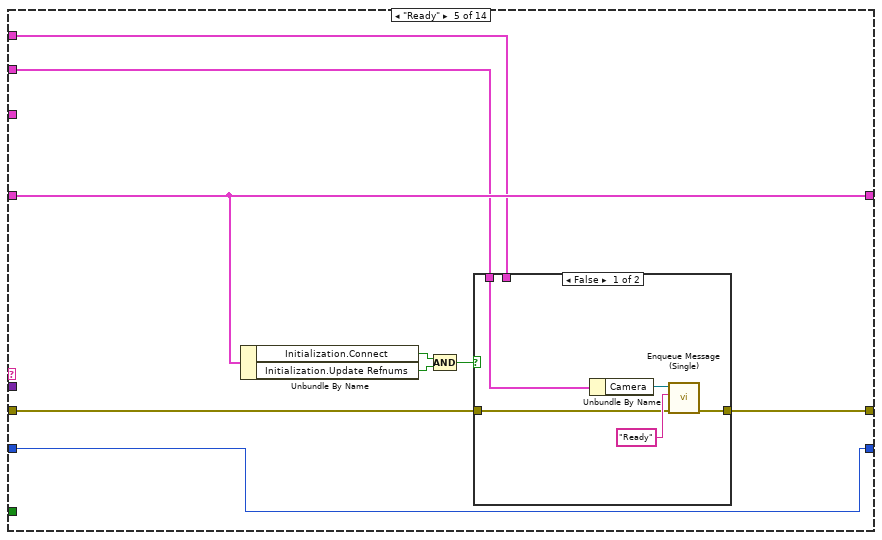
[diagram p7: hidden frame]
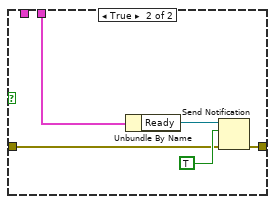
[diagram p8: hidden frame]
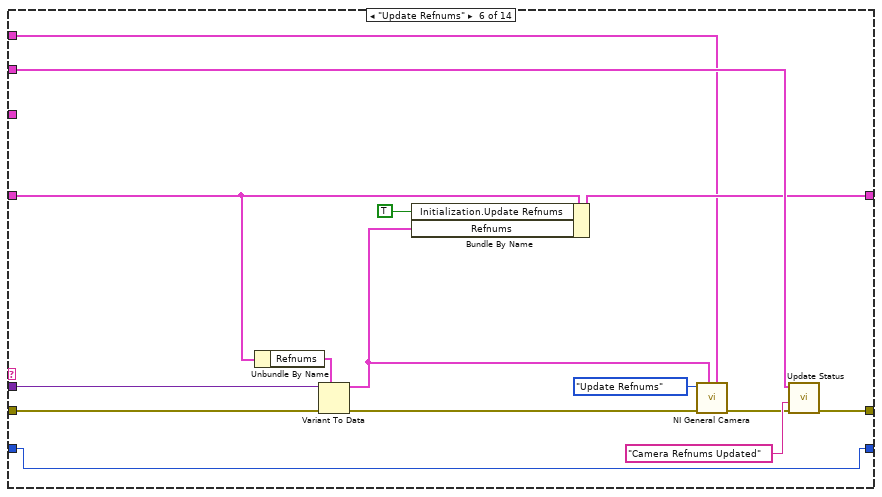
[diagram p9: hidden frame]
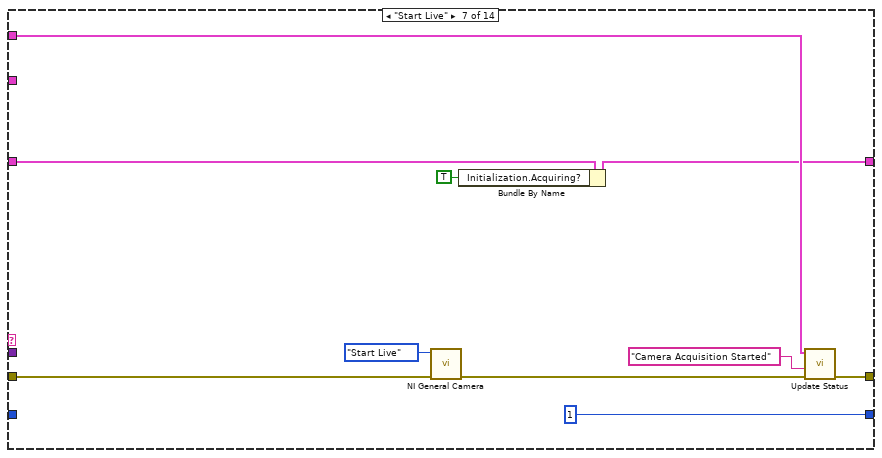
[diagram p10: hidden frame]
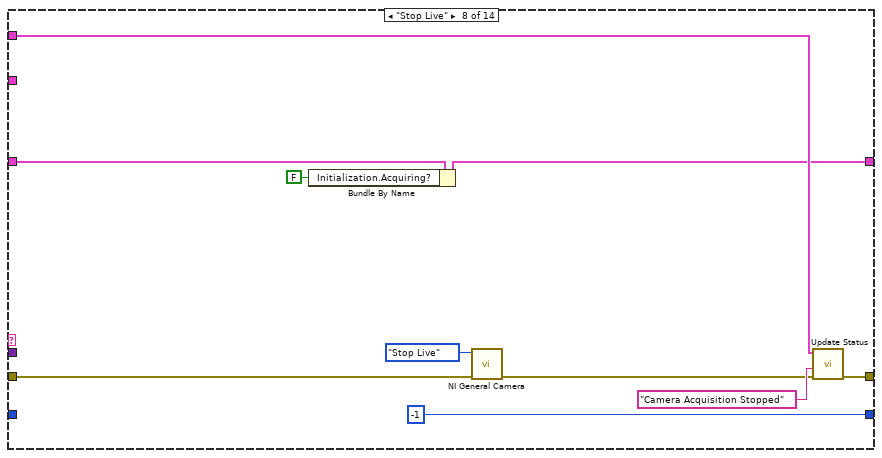
[diagram p11: hidden frame]
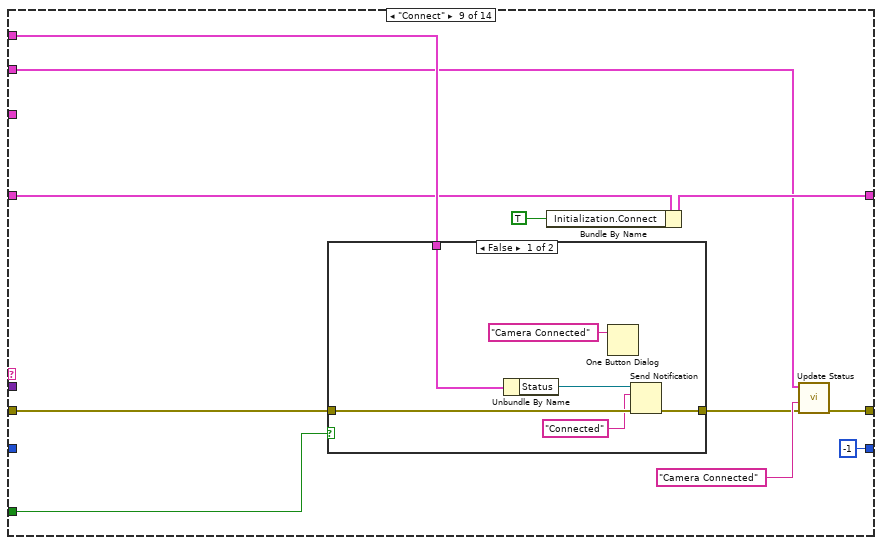
[diagram p12: hidden frame]
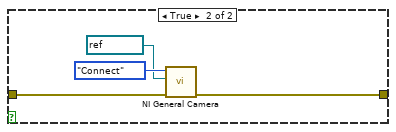
[diagram p13: hidden frame]
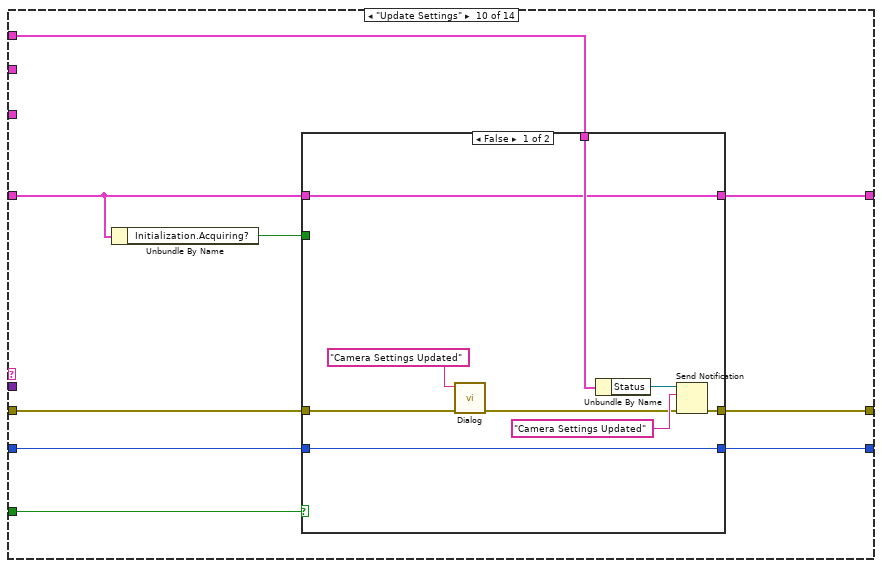
[diagram p14: hidden frame]
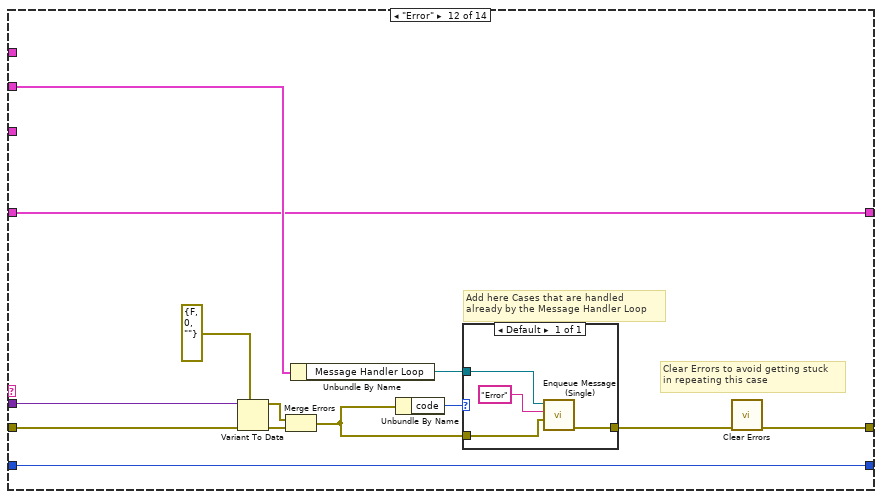
[diagram p17: hidden frame]
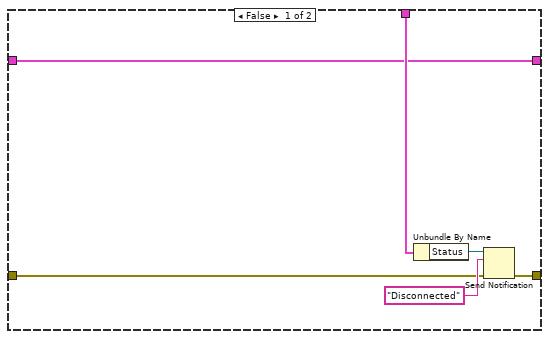
[diagram p18: hidden frame]
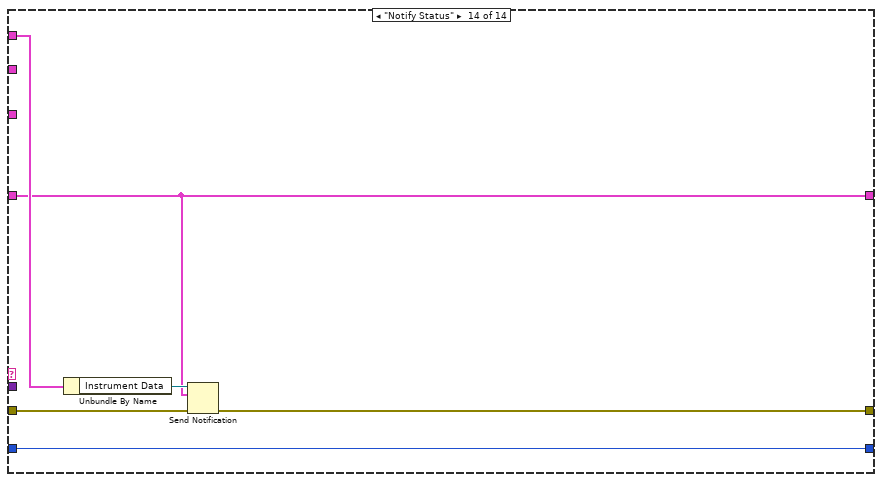
[diagram p20: hidden frame]
diagram:
  w3 = -1  # Frame Rate
  # "LICENSED MATERIALS – PROPERTY OF IBM\nCopyright IBM Corp. 2016,\nALL RIGHTS RESERVED"
  n1 = call "Camera Data.vi"() -> ("Camera Data"=w5:T58)
  n2 = while "Queued Message Handler for Camera" {
    tunnel: "error in" -> [w11]
    tunnel: [w23] -> w1
    tunnel: "Message Queues out" -> [w26]
    tunnel: "Notifiers" -> [w17]
    tunnel: "IBM OptoElectroMechanics Configuration" -> [w22]
    shift-right: [w18] -> _
    shift-left: w5 -> [w19]
    shift-right: [w9] -> _
    shift-left: w3 -> [w8]
    stop <- w25 stop-if-true
    # "Configurations"
    # "Notifiers"
    # "Message Queues"
    n3 = Unbundle By Name(w26) -> ("Camera"=w15:refnum<queue>)
    n4 = Unbundle By Name(w17) -> ("Camera"=w16:T51)
    n5 = Unbundle By Name(w22) -> ("Camera"=w21:T22)
    n6 = call "Dequeue Message With Timeout.vi"("error in (no error)"=w11, "Timeout in ms (-1)"=w8, "Queue In"=w15) -> ("error out"=w12:errorcluster, "Message Data"=w13:variant, "Message"=w14:string, "timed out?"=w10:bool)  [unwired: 4 in, 1 out]
    n7 = case shown="False" w10 {
      tunnel: w26 -> [w39 _]
      tunnel: [w38 _] -> w25
      tunnel: [w37 w251] -> w24
      tunnel: w21 -> [w36 _]
      tunnel: "Used functions" -> [w35 _]
      tunnel: w19 -> [w34 w250]
      tunnel: [w33 w250] -> w18
      tunnel: w16 -> [w32 _]
      tunnel: w14 -> [w31 _]
      tunnel: w13 -> [w30 _]
      tunnel: w12 -> [w29 w252]
      tunnel: w8 -> [w28 w253]
      tunnel: [w27 w253] -> w9
      frame False {
        n8 = case shown="\"Exit\"" w31 {
          selector: w31 -> [w43 _ _ _ _ _ _ _ _ _ _ _ _ _]
          tunnel: w29 -> [_ w57 w64 w78 w93 w121 w124 w134 w148 w165 w185 w197 w205 w248]
          tunnel: [w42 w52 w65 w86 w91 w120 w132 w142 w144 w164 w185 w192 w212 w247] -> w37
          tunnel: w30 -> [_ _ _ _ _ w122 _ _ _ _ _ w190 _ _]
          tunnel: w39 -> [_ w60 w66 w88 w92 w118 w130 w140 w146 _ _ w198 w217 _]
          tunnel: w32 -> [_ _ _ _ w90 w111 _ _ w152 w169 _ _ w210 w246]
          tunnel: [_ _ _ _ _ _ _ _ _ _ _ _ TRUE ("Priority Message? (F)") _] -> w38
          tunnel: w36 -> [_ w51 _ _ _ _ _ _ _ _ _ _ _ _]
          tunnel: w34 -> [w41 w59 w63 w84 w95 w115 w127 w139 w150 w170 w186 w189 w215 w243]
          tunnel: w35 -> [_ _ _ _ _ _ _ _ w153 w172 _ _ w218 _]
          tunnel: [w41 w50 w63 w84 w95 w117 w129 w138 w151 w171 w186 w189 w214 w243] -> w33
          tunnel: w28 -> [w40 w49 w61 w81 w89 w113 _ _ _ w166 w187 w188 _ w244]
          tunnel: [w40 w49 w61 w81 w89 w113 1 ("Frame Rate") -1 -1 ("Frame Rate") w167 w187 w188 -1 w244] -> w27
          frame Default {
            # "The Defualt Case run if there is a message that isn't defined in any of the other cases.\nOutput a program error"
            n9 = Format Into String(format string="The invalid message string \"%s\" was  received in the Camera Loop", w43) -> (resulting string=w45:string)  [unwired: 2 in, 1 out]
            n10 = call <vilib>:"Error Cluster From Error Code.vi"("error message (\"\")"=w45, "error code (0)"=5001) -> ("error out"=w42:errorcluster)  [unwired: 2 in, 5 out]
          }
          frame "Initialize" {
            n11 = Unbundle By Name(w60) -> ("Camera"=w48:refnum<queue>, "Message Handler Loop"=w53:refnum<queue>)
            n12 = call "Enqueue Message (Single).vi"("error in (no error)"=w57, "Message"="Camera - Update Refnums", "Message Queue"=w53) -> ("error out"=w55:errorcluster)  [unwired: 1 in, 7 out]
            n13 = call "Enqueue Message (Single).vi"("error in (no error)"=w55, "Message Data"=w51, "Message"="Camera - Set UI", "Message Queue"=w53) -> ("error out"=w47:errorcluster)  [unwired: 7 out]
            n14 = call "Enqueue Message (Single).vi"("error in (no error)"=w47, "Message"="Check if Refnum Update", "Message Queue"=w48) -> ("error out"=w52:errorcluster)  [unwired: 1 in, 7 out]
            n15 = Bundle By Name(cluster=w59, "Configuration"=w51) -> (w50:T58)
          }
          frame "Check if Refnum Update" {
            n16 = Unbundle By Name(w63) -> ("Initialization.Update Refnums"=w62:bool)
            n17 = case shown="False" w62 {
              tunnel: w66 -> [w71 w76]
              tunnel: [w68 w73] -> w65
              tunnel: w64 -> [w67 w72]
              frame True {
                n18 = Unbundle By Name(w71) -> ("Camera"=w69:refnum<queue>)
                n19 = call "Enqueue Message (Single).vi"("error in (no error)"=w67, "Message"="Continue Initialize", "Message Queue"=w69) -> ("error out"=w68:errorcluster)  [unwired: 1 in, 7 out]
              }
              frame False {
                n20 = Unbundle By Name(w76) -> ("Camera"=w74:refnum<queue>)
                n21 = call "Enqueue Message (Single).vi"("error in (no error)"=w72, "Message"="Check if Refnum Update", "Message Queue"=w74) -> ("error out"=w73:errorcluster)  [unwired: 1 in, 7 out]
              }
            }
          }
          frame "Continue Initialize" {
            n22 = Unbundle By Name(w84) -> ("Configuration"=w83:T22)
            n23 = Unbundle By Name(w88) -> ("Camera"=w79:refnum<queue>)
            n24 = call "Enqueue Message (Single).vi"("error in (no error)"=w78, "Message"="Connect", "Message Queue"=w79) -> ("error out"=w77:errorcluster)  [unwired: 1 in, 7 out]
            n25 = call "Enqueue Message (Single).vi"("error in (no error)"=w77, "Message Data"=w83, "Message"="Update Settings", "Message Queue"=w79) -> ("error out"=w82:errorcluster)  [unwired: 7 out]
            n26 = call "Enqueue Message (Single).vi"("error in (no error)"=w82, "Message"="Ready", "Message Queue"=w79) -> ("error out"=w86:errorcluster)  [unwired: 1 in, 7 out]
          }
          frame "Ready" {
            n27 = Unbundle By Name(w95) -> ("Initialization.Connect"=w96:bool, "Initialization.Update Refnums"=w94:bool)
            n28 = Compound Arithmetic op=AND(w96, w94) -> (w97:bool)
            n29 = case shown="False" w97 {
              tunnel: [w100 w105] -> w91
              tunnel: w93 -> [w99 w104]
              tunnel: w92 -> [w98 _]
              tunnel: w90 -> [_ w103]
              frame False {
                n30 = Unbundle By Name(w98) -> ("Camera"=w102:refnum<queue>)
                n31 = call "Enqueue Message (Single).vi"("error in (no error)"=w99, "Message"="Ready", "Message Queue"=w102) -> ("error out"=w100:errorcluster)  [unwired: 1 in, 7 out]
              }
              frame True {
                n32 = Unbundle By Name(w103) -> ("Ready"=w106:refnum<notifier>)
                n33 = Send Notification(notification=TRUE, notifier=w106, error in (no error)=w104) -> (error out=w105:errorcluster)  [unwired: 1 out]
              }
            }
          }
          frame "Update Refnums" {
            n34 = Unbundle By Name(w115) -> ("Refnums"=w114:T59)
            n35 = Variant To Data(error in=w121, type=w114, Variant=w122) -> (data=w112:T59, error out=w109:errorcluster)
            n36 = Bundle By Name(cluster=w115, "Initialization.Update Refnums"=TRUE, "Refnums"=w112) -> (w117:T58)
            n37 = call "NI General Camera.vi"("Camera Notifiers"=w111, "Refnums"=w112, "error in (no error)"=w109, "Function"=NI_Camera_Functions."Update Refnums") -> ("error out"=w108:errorcluster)  [unwired: 4 in, 3 out]
            n38 = call "Update Status.vi"("error in"=w108, "String"="Camera Refnums Updated" ("button name (\"OK\")"), "Message Queues out"=w118) -> ("error out"=w120:errorcluster)  [unwired: 8 out]
          }
          frame "Start Live" {
            n39 = call "NI General Camera.vi"("error in (no error)"=w124, "Function"=NI_Camera_Functions."Start Live") -> ("error out"=w123:errorcluster)  [unwired: 6 in, 3 out]
            n40 = Bundle By Name(cluster=w127, "Initialization.Acquiring?"=TRUE ("Initialization.Acquiring")) -> (w129:T58)
            n41 = call "Update Status.vi"("error in"=w123, "String"="Camera Acquisition Started" ("button name (\"OK\")"), "Message Queues out"=w130) -> ("error out"=w132:errorcluster)  [unwired: 8 out]
          }
          frame "Stop Live" {
            n42 = Bundle By Name(cluster=w139, "Initialization.Acquiring?"=FALSE ("Initialization.Acquiring")) -> (w138:T58)
            n43 = call "NI General Camera.vi"("error in (no error)"=w134, "Function"=NI_Camera_Functions."Stop Live") -> ("error out"=w133:errorcluster)  [unwired: 6 in, 3 out]
            n44 = call "Update Status.vi"("error in"=w133, "String"="Camera Acquisition Stopped" ("button name (\"OK\")"), "Message Queues out"=w140) -> ("error out"=w142:errorcluster)  [unwired: 8 out]
          }
          frame "Connect" {
            n45 = case shown="False" w153 {
              tunnel: w148 -> [w157 w162]
              tunnel: [w156 w160] -> w145
              tunnel: w152 -> [w159 _]
              frame False {
                n46 = Unbundle By Name(w159) -> ("Status"=w158:refnum<notifier>)
                n47 = One Button Dialog(message="Camera Connected" ("button name (\"OK\")")) -> ()  [unwired: 2 out]
                n48 = Send Notification(notification="Connected", notifier=w158, error in (no error)=w157) -> (error out=w156:errorcluster)  [unwired: 1 out]
              }
              frame True {
                n49 = call "NI General Camera.vi"("error in (no error)"=w162, "Camera Name"=refnum<k21> "cam0", "Function"=NI_Camera_Functions."Connect") -> ("error out"=w160:errorcluster)  [unwired: 5 in, 3 out]
              }
            }
            n50 = Bundle By Name(cluster=w150, "Initialization.Connect"=TRUE ("Initialization.Update Visa Session")) -> (w151:T58)
            n51 = call "Update Status.vi"("error in"=w145, "String"="Camera Connected" ("button name (\"OK\")"), "Message Queues out"=w146) -> ("error out"=w144:errorcluster)  [unwired: 8 out]
          }
          frame "Update Settings" {
            n52 = Unbundle By Name(w170) -> ("Initialization.Acquiring?"=w168:bool)
            n53 = case shown="False" w172 {
              tunnel: w165 -> [w178 w184]
              tunnel: [w176 w184] -> w164
              tunnel: w170 -> [w174 w183]
              tunnel: [w174 w183] -> w171
              tunnel: w169 -> [w175 _]
              tunnel: w168 -> [_ _]
              tunnel: [w173 w182] -> w167
              tunnel: w166 -> [w173 w182]
              frame False {
                n54 = call "Dialog.vi"("error in (no error)"=w178, "message"="Camera Settings Updated" ("button name (\"OK\")")) -> ("error out"=w177:errorcluster)  [unwired: 1 in, 8 out]
                n55 = Unbundle By Name(w175) -> ("Status"=w179:refnum<notifier>)
                n56 = Send Notification(notification="Camera Settings Updated", notifier=w179, error in (no error)=w177) -> (error out=w176:errorcluster)  [unwired: 1 out]
              }
              frame True {
              }
            }
          }
          frame "Popup" {
          }
          frame "Error" {
            # "Clear Errors to avoid getting stuck \nin repeating this case"
            # "Add here Cases that are handled \nalready by the Message Handler Loop"
            n57 = Variant To Data(error in=w197, type=errorcluster {"status"=FALSE, "code"=0, "source"=""} ("error out"), Variant=w190) -> (data=w196:errorcluster, error out=w195:errorcluster)
            n58 = Merge Errors(w196, w195) -> (w194:errorcluster)
            n59 = Unbundle By Name(w198) -> ("Message Handler Loop"=w200:refnum<queue>)
            n60 = Unbundle By Name(w194) -> ("code"=w191:i32)
            n61 = case shown="Default" w191 {
              tunnel: w200 -> [w204]
              tunnel: w194 -> [w202]
              tunnel: [w201] -> w193
              frame Default {
                n62 = call "Enqueue Message (Single).vi"("Message Data"=w202, "Message"="Error", "Message Queue"=w204) -> ("error out"=w201:errorcluster)  [unwired: 1 in, 7 out]
              }
            }
            n63 = call <vilib>:"Clear Errors.vi"("error in (no error)"=w193) -> ("error out"=w192:errorcluster)  [unwired: 1 in, 5 out]
          }
          frame "Exit" {
            w206 = TRUE ("Priority Message? (F)")
            # "Stop the VI"
            n64 = case shown="True" w218 {
              tunnel: w205 -> [w225 w229]
              tunnel: [w224 w230] -> w208
              tunnel: w210 -> [w223 _]
              tunnel: w215 -> [w222 w233]
              tunnel: [w222 w234] -> w214
              frame False {
                n65 = Unbundle By Name(w223) -> ("Status"=w226:refnum<notifier>)
                n66 = Send Notification(notification="Disconnected", notifier=w226, error in (no error)=w225) -> (error out=w224:errorcluster)  [unwired: 1 out]
              }
              frame True {
                n67 = Unbundle By Name(w233) -> ("Initialization.Acquiring?"=w232:bool)
                n68 = case shown="True" w232 {
                  tunnel: w229 -> [w235 w238]
                  tunnel: w233 -> [w236 w242]
                  tunnel: [w236 w241] -> w234
                  tunnel: [w235 w237] -> w228
                  frame False {
                  }
                  frame True {
                    n69 = Bundle By Name(cluster=w242, "Initialization.Acquiring?"=FALSE) -> (w241:T58)
                    n70 = call "NI General Camera.vi"("error in (no error)"=w238, "Function"=NI_Camera_Functions."Stop Live") -> ("error out"=w237:errorcluster)  [unwired: 6 in, 3 out]
                  }
                }
                n71 = call "NI General Camera.vi"("error in (no error)"=w228, "Function"=NI_Camera_Functions."Disconnect") -> ("error out"=w230:errorcluster)  [unwired: 6 in, 3 out]
              }
            }
            n72 = Unbundle By Name(w217) -> ("Camera"=w221:refnum<queue>)
            n73 = Unbundle By Name(w210) -> ("Ready"=w209:refnum<notifier>)
            n74 = Unbundle By Name(w210) -> ("Exit"=w220:refnum<notifier>)
            n75 = Send Notification(notification=w206, notifier=w209, error in (no error)=w208) -> (error out=w207:errorcluster)  [unwired: 1 out]
            n76 = Send Notification(notification=w206, notifier=w220, error in (no error)=w208) -> (error out=w211:errorcluster)  [unwired: 1 out]
            n77 = Release Queue(queue=w221, error in (no error)=w208) -> (error out=w213:errorcluster)  [unwired: 3 out]
            n78 = Merge Errors(w207, w211, w213) -> (w212:errorcluster)
          }
          frame "Notify Status" {
            n79 = Unbundle By Name(w246) -> ("Instrument Data"=w245:refnum<notifier>)
            n80 = Send Notification(notification=w243, notifier=w245, error in (no error)=w248) -> (error out=w247:errorcluster)  [unwired: 1 out]
          }
        }
      }
      frame True {
        n81 = Unbundle By Name(w250) -> ("Initialization.Acquiring?"=w249:bool)
        n82 = case shown="True" w249 {
          tunnel: w252 -> [w254 w256]
          tunnel: [w254 w255] -> w251
          frame False {
          }
          frame True {
            n83 = call "NI General Camera.vi"("error in (no error)"=w256, "Function"=NI_Camera_Functions."Acquire") -> ("error out"=w255:errorcluster)  [unwired: 6 in, 3 out]
          }
        }
      }
    }
    n84 = call "Message Handling Loop.vi"("error in (no error)"=w24, "Message Queue"=w15) -> ("dup error in"=w23:errorcluster)  [unwired: 9 out]
  }
  "error out" <- w1
